vi "Acquire.vi"(0 "Hardware Resources in":T9, 1 "Config Data":T1, 2 "Data Notifier":refnum<notifier>, 3 "Data Queue":refnum<queue>, 5 "error in (no error)":errorcluster, 6 "Message Queues":T7, 7 "Acquisition Metrics in":T8) -> (13 "Acquisition Metrics out":T8, 14 "Hardware Resources out":T9, 19 "error out":errorcluster)   [LabVIEW 2026, in "Acquisition.lvlib"]
doc: "Perform the acquisition. Replace the contents of this diagram with calls to acquisition hardware."
uses:
  Acquisition.lvlib
  Controls/Hardware Configuration.ctl
  Controls/Machine_State_Buffer.ctl
  Controls/Acquisition Metrics.ctl
  Support/Message Queue/All Message Queues.ctl
  Support/Message Queue/Message Cluster.ctl
  Controls/Vibration_Monitor_Config.ctl
  Controls/Vibration_Profile.ctl
  Controls/System_Settings.ctl
  Controls/Options.ctl
  Controls/Relay_Profile.ctl
  Controls/RPM_Profile.ctl
  <vilib>/DAQmx/read.llb/DAQmx Read (Analog 1D Wfm NChan NSamp).vi
  <vilib>/DAQmx/miscellaneous.llb/DAQmx Fill In Error Info.vi
  Support/Message Queue/Enqueue Message (Single).vi
  support/Message Queue/Message Queue.lvlib
  <userlib>/_OpenG.lib/error/error.llb/openg_error.lvlib
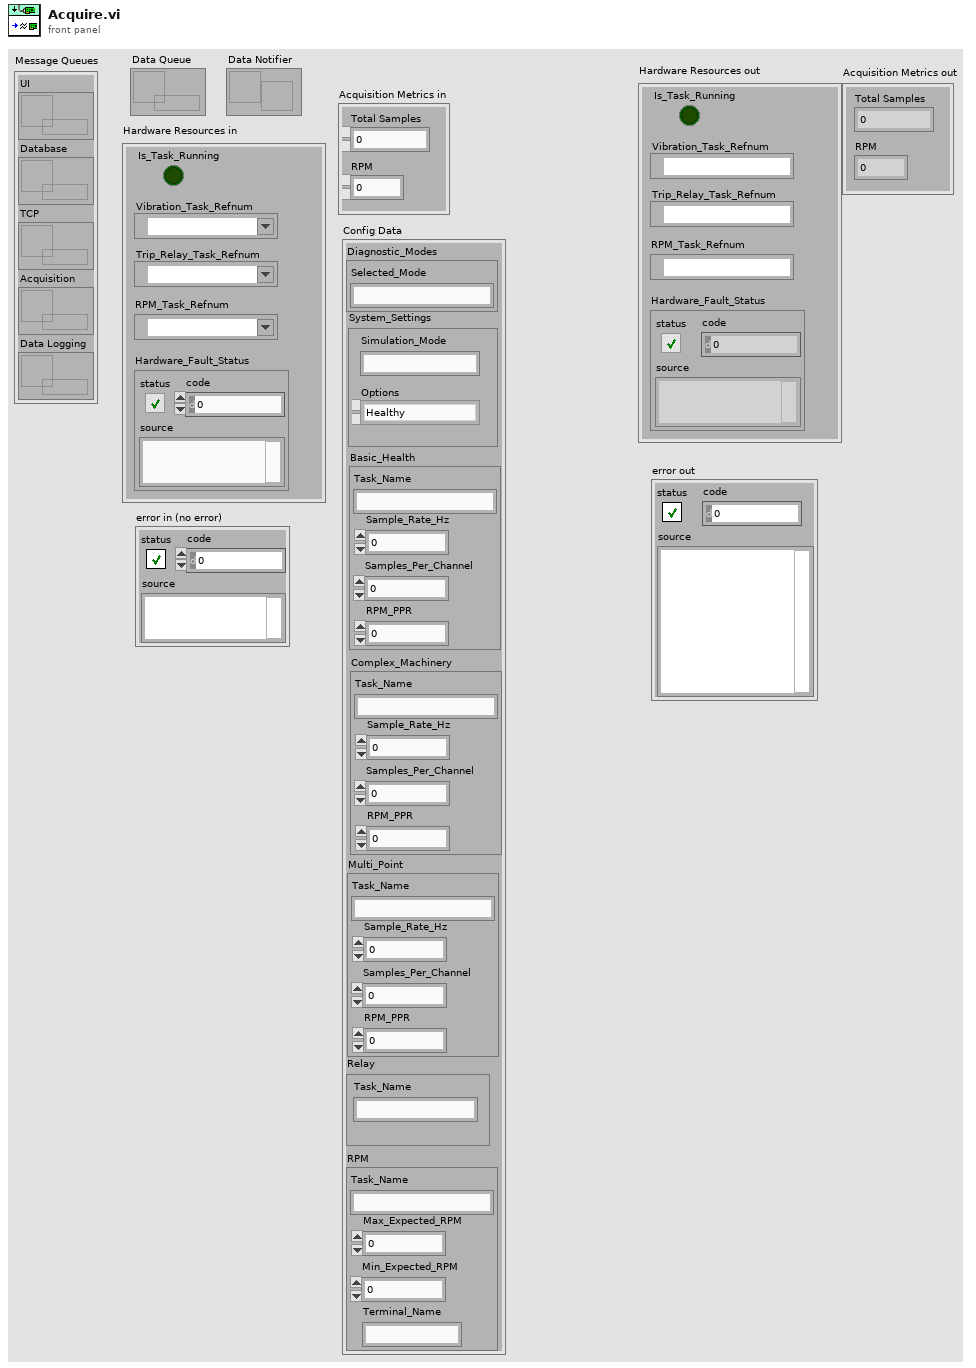
[diagram p1: front panel]
types:
  T1 = typedef "Vibration_Monitor_Config.ctl" = cluster{"Diagnostic_Modes":cluster{"Selected_Mode":string}, "Basic_Health":T2, "Complex_Machinery":T2, "Multi_Point":T2, "System_Settings":T3, "Relay":T5, "RPM":T6}
  T2 = typedef "Vibration_Profile.ctl" = cluster{"Task_Name":string, "Sample_Rate_Hz":dbl, "Samples_Per_Channel":i32, "RPM_PPR ":dbl}
  T3 = typedef "System_Settings.ctl" = cluster{"Simulation_Mode ":string, "Options":T4}
  T4 = typedef "Options.ctl" = enum16{"Healthy", "Unbalance_Alert", "Bearing_Fault_Critical", "Sweep_Test"}
  T5 = typedef "Relay_Profile.ctl" = cluster{"Task_Name":string}
  T6 = typedef "RPM_Profile.ctl" = cluster{"Task_Name":string, "Max_Expected_RPM":dbl, "Min_Expected_RPM":dbl, "Terminal_Name":string}
  T7 = typedef "Message Queue.lvlib/All Message Queues.ctl" = cluster{"UI":refnum<queue>, "Database":refnum<queue>, "TCP":refnum<queue>, "Acquisition":refnum<queue>, "Data Logging":refnum<queue>}
  T8 = typedef "Acquisition.lvlib/Acquisition Metrics.ctl" = cluster{"Total_Samples":i64, "rpm":dbl}
  T9 = typedef "Acquisition.lvlib/Hardware Configuration.ctl" = cluster{"Vibration_Task_Refnum":refnum<k21>, "Hardware_Fault_Status":errorcluster, "Trip_Relay_Task_Refnum":refnum<k21>, "RPM_Task_Refnum":refnum<k21>, "Is_Task_Running":bool}
  T10 = typedef "Machine_State_Buffer.ctl" = cluster{"Waveforms":waveform(dbl)[], "Acquisition Metrics":T8}
  T11 = typedef "Acquisition.lvlib/Alarms.ctl" = cluster{"Excellent":bool, "Healthy":bool, "Predictive Alarm":bool, "Hardware Trip":bool}
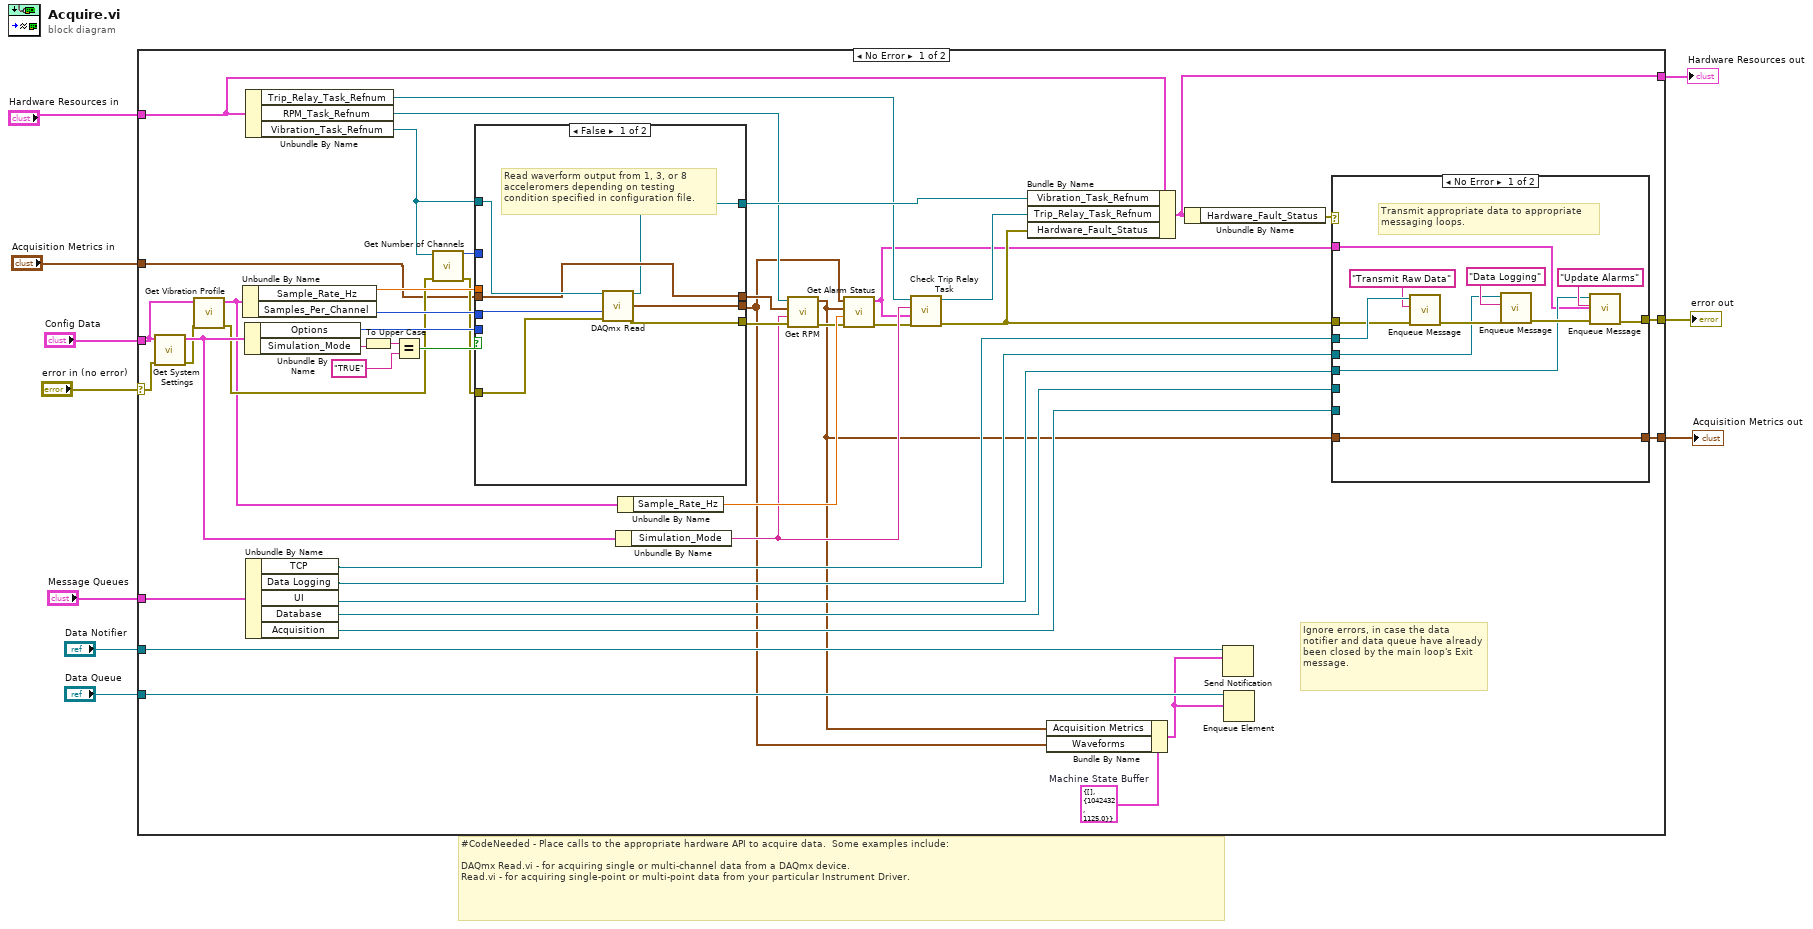
[diagram p0: block diagram]
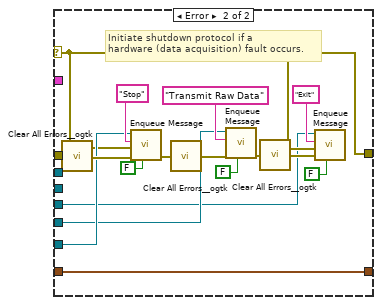
[diagram p2: hidden frame]
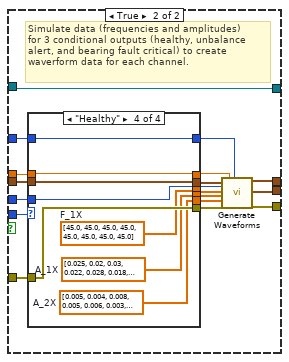
[diagram p3: hidden frame]
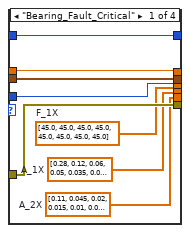
[diagram p4: hidden frame]
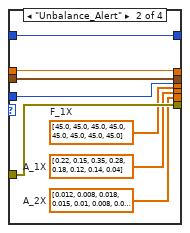
[diagram p5: hidden frame]
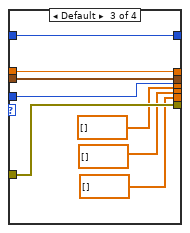
[diagram p6: hidden frame]
diagram:
  # "#CodeNeeded - Place calls to the appropriate hardware API to acquire data.  Some examples include:\n\nDAQmx Read.vi - for acquiring single or multi-channel data from a DAQmx device.\nRead.vi - for acquiring single-point or multi-point data from your particular Instrument Driver."
  n1 = case shown="No Error" "error in (no error)" {
    selector: "error in (no error)" -> [w30 w144]
    tunnel: [w34 w144] -> w9
    tunnel: "Hardware Resources in" -> [w40 w145]
    tunnel: [w33 w145] -> w7
    tunnel: "Data Notifier" -> [w56 _]
    tunnel: "Data Queue" -> [w55 _]
    tunnel: "Acquisition Metrics in" -> [w26 w143]
    tunnel: "Message Queues" -> [w39 _]
    tunnel: "Config Data" -> [w27 _]
    tunnel: [w15 w143] -> w1
    frame No Error {
      w14 = T10 {"Waveforms"=[], "Acquisition Metrics"={"Total_Samples"=1042432, "rpm"=1125.0}}  # Machine State Buffer
      # "Ignore errors, in case the data notifier and data queue have already been closed by the main loop's Exit message."
      n2 = call "Get System Settings.vi"("error in (no error)"=w30, "Config Data"=w27) -> ("error out"=w29:errorcluster, "System_Settings"=w31:T3)  [unwired: 8 in]
      n3 = call "Get Vibration Profile.vi"("error in (no error)"=w29, "Config Data"=w27) -> ("error out"=w28:errorcluster, "Active Vibration Profile"=w25:T2)  [unwired: 8 in]
      n4 = Unbundle By Name(w25) -> ("Sample_Rate_Hz"=w48:dbl, "Samples_Per_Channel"=w54:i32)
      n5 = Unbundle By Name(w31) -> ("Options"=w49:T4, "Simulation_Mode"=w53:string)
      n6 = Unbundle By Name(w40) -> ("Trip_Relay_Task_Refnum"=w23:refnum<k21>, "RPM_Task_Refnum"=w22:refnum<k21>, "Vibration_Task_Refnum"=w45:refnum<k21>)
      n7 = Unbundle By Name(w39) -> ("TCP"=w38:refnum<queue>, "Data Logging"=w37:refnum<queue>, "UI"=w36:refnum<queue>, "Database"=w35:refnum<queue>, "Acquisition"=w32:refnum<queue>)
      n8 = To Upper Case(1:w53) -> (0:w52:string)
      n9 = Equal?(x=w52, y="TRUE") -> (x = y?=w50:bool)
      n10 = call "Get Number of Channels.vi"("error in (no error)"=w28, "Refnum in"=w45) -> ("error out"=w44:errorcluster, "Number of Channels"=w46:i32)  [unwired: 8 in]
      n11 = case shown="False" w50 {
        tunnel: w44 -> [w91 w109]
        tunnel: w54 -> [w92 w108]
        tunnel: [w90 w101] -> w20
        tunnel: w49 -> [_ w110]
        tunnel: w48 -> [_ w100]
        tunnel: w45 -> [w88 w107]
        tunnel: [w89 w97] -> w12
        tunnel: [w86 w107] -> w47
        tunnel: w46 -> [_ w106]
        tunnel: w26 -> [w87 w99]
        tunnel: [w87 w96] -> w21
        frame False {
          # "Read waverform output from 1, 3, or 8 \nacceleromers depending on testing \ncondition specified in configuration file."
          n12 = call-poly <vilib>:"DAQmx Read.vi"("task/channels in"=w88, "number of samples per channel"=w92, "error in"=w91) -> ("task out"=w86:refnum<k21>, "data"=w89:waveform(dbl)[], "error out"=w90:errorcluster)  [unwired: 10 in]
        }
        frame True {
          # "Simulate data (frequencies and amplitudes)\nfor 3 conditional outputs (healthy, unbalance \nalert, and bearing fault critical) to create\nwaverform data for each channel."
          n13 = case shown="\"Healthy\"" w110 {
            tunnel: w109 -> [w118 w126 w132 w142]
            tunnel: w108 -> [w117 w125 w133 w141]
            tunnel: w106 -> [w116 w124 w134 w140]
            tunnel: [w118 w126 w132 w142] -> w105
            tunnel: [w117 w125 w133 w141] -> w104
            tunnel: [w115 w123 w131 w139] -> w103
            tunnel: [w116 w124 w134 w140] -> w102
            tunnel: w100 -> [w115 w123 w131 w139]
            tunnel: w99 -> [w114 w122 w130 w138]
            tunnel: [w114 w122 w130 w138] -> w98
            tunnel: [w113 w121 dbl[] [] ("Amplitudes") w137] -> w95
            tunnel: [w112 w120 dbl[] [] ("Frequencies") w136] -> w94
            tunnel: [w111 w119 dbl[] [] ("Frequencies") w135] -> w93
            frame "Bearing_Fault_Critical" {
              w111 = dbl[] [0.11, 0.045, 0.02, 0.015, 0.01, 0.008, 0.008, 0.005]  # A_2X
              w112 = dbl[] [0.28, 0.12, 0.06, 0.05, 0.035, 0.025, 0.03, 0.02]  # A_1X
              w113 = dbl[] [45.0, 45.0, 45.0, 45.0, 45.0, 45.0, 45.0, 45.0]  # F_1X
            }
            frame "Unbalance_Alert" {
              w121 = dbl[] [45.0, 45.0, 45.0, 45.0, 45.0, 45.0, 45.0, 45.0]  # F_1X
              w119 = dbl[] [0.012, 0.008, 0.018, 0.015, 0.01, 0.008, 0.01, 0.003]  # A_2X
              w120 = dbl[] [0.22, 0.15, 0.35, 0.28, 0.18, 0.12, 0.14, 0.04]  # A_1X
            }
            frame Default {
            }
            frame "Healthy" {
              w135 = dbl[] [0.005, 0.004, 0.008, 0.005, 0.006, 0.003, 0.009, 0.002]  # A_2X
              w137 = dbl[] [45.0, 45.0, 45.0, 45.0, 45.0, 45.0, 45.0, 45.0]  # F_1X
              w136 = dbl[] [0.025, 0.02, 0.03, 0.022, 0.028, 0.018, 0.035, 0.015]  # A_1X
            }
          }
          n14 = call "Generate Waveforms.vi"("Acquisition Metrics in"=w98, "Samples Per Channel"=w104, "F_1X"=w95, "A_1X"=w94, "A_2X"=w93, "error in (no error)"=w105, "Sample Rate Hz"=w103, "Number of Channels"=w102) -> ("Acquisition Metrics out"=w96:T8, "Waveforms"=w97:waveform(dbl)[], "error out"=w101:errorcluster)  [unwired: 9 in]
        }
      }
      n15 = Unbundle By Name(w31) -> ("Simulation_Mode"=w19:string)
      n16 = Unbundle By Name(w25) -> ("Sample_Rate_Hz"=w24:dbl)
      n17 = call "Get RPM.vi"("error in (no error)"=w20, "Simulation Mode"=w19, "Acquisition Metrics in"=w21, "task/channels in"=w22) -> ("error out"=w18:errorcluster, "Acquisition Metrics out"=w13:T8)  [unwired: 6 in]
      n18 = call "Get Alarm Status.vi"("error in (no error)"=w18, "Sample Rate Hz"=w24, "Acquisition Metrics in"=w13, "data"=w12) -> ("error out"=w17:errorcluster, "Alarms"=w16:T11)  [unwired: 6 in]
      n19 = call "Check Trip Relay Task.vi"("error in (no error)"=w17, "Alarms"=w16, "Simulation Mode"=w19, "task/channels in"=w23) -> ("error out"=w41:errorcluster, "task out"=w43:refnum<k21>)  [unwired: 6 in]
      n20 = Bundle By Name(cluster=w40, "Vibration_Task_Refnum"=w47, "Trip_Relay_Task_Refnum"=w43, "Hardware_Fault_Status"=w41) -> (w33:T9)
      n21 = Bundle By Name(cluster=w14, "Acquisition Metrics"=w13, "Waveforms"=w12) -> (w11:T10)
      n22 = Unbundle By Name(w33) -> ("Hardware_Fault_Status"=w42:errorcluster)
      n23 = Send Notification(notification=w11, notifier=w56) -> ()  [unwired: 1 in, 2 out]
      n24 = Enqueue Element(queue=w55, element=w11) -> ()  [unwired: 2 in, 3 out]
      n25 = case shown="No Error" w42 {
        selector: w42 -> [_ w71]
        tunnel: w38 -> [w64 _]
        tunnel: w37 -> [w63 _]
        tunnel: w36 -> [w62 w70]
        tunnel: w41 -> [w61 w82]
        tunnel: w35 -> [_ w72]
        tunnel: [w60 w71] -> w34
        tunnel: w32 -> [_ w73]
        tunnel: w16 -> [w59 _]
        tunnel: w13 -> [w58 w69]
        tunnel: [w58 w69] -> w15
        frame No Error {
          # "Transmit appropriate data to appropriate \nmessaging loops."
          n26 = call-poly "Enqueue Message.vi"("error in (no error)"=w61, "Message"="Transmit Raw Data", "Message Queue"=w64) -> ("error out"=w67:errorcluster)  [unwired: 7 in, 1 out]
          n27 = call-poly "Enqueue Message.vi"("error in (no error)"=w67, "Message"="Data Logging", "Message Queue"=w63) -> ("error out"=w65:errorcluster)  [unwired: 7 in, 1 out]
          n28 = call-poly "Enqueue Message.vi"("error in (no error)"=w65, "Message Data"=w59, "Message"="Update Alarms", "Message Queue"=w62) -> ("error out"=w60:errorcluster)  [unwired: 6 in, 1 out]
        }
        frame Error {
          # "Initiate shutdown protocol if a \nhardware (data acquisition) fault occurs."
          n29 = call <userlib>:"Clear All Errors__ogtk.vi"("Error In"=w82) -> ("Error Out"=w81:errorcluster)  [unwired: 3 in]
          n30 = call-poly "Enqueue Message.vi"("Priority Message? (F)"=FALSE, "error in (no error)"=w81, "Message Data"=w71, "Message"="Stop", "Message Queue"=w73) -> ("error out"=w80:errorcluster)  [unwired: 5 in, 1 out]
          n31 = call <userlib>:"Clear All Errors__ogtk.vi"("Error In"=w80) -> ("Error Out"=w76:errorcluster)  [unwired: 3 in]
          n32 = call-poly "Enqueue Message.vi"("Priority Message? (F)"=FALSE, "error in (no error)"=w76, "Message"="Transmit Raw Data", "Message Queue"=w72) -> ("error out"=w75:errorcluster)  [unwired: 6 in, 1 out]
          n33 = call <userlib>:"Clear All Errors__ogtk.vi"("Error In"=w75) -> ("Error Out"=w74:errorcluster)  [unwired: 3 in]
          n34 = call-poly "Enqueue Message.vi"("Priority Message? (F)"=FALSE, "error in (no error)"=w74, "Message Data"=w71, "Message"="Exit", "Message Queue"=w70) -> ()  [unwired: 5 in, 2 out]
        }
      }
    }
    frame Error {
    }
  }
  "Hardware Resources out" <- w7
  "error out" <- w9
  "Acquisition Metrics out" <- w1
